vi "setMeasurement.vi"(1 "Measure":T1, 2 "Channel":T2) -> (0 "String":string)   [LabVIEW 2017]
uses:
  controls/Channel.ctl
  controls/Measure.ctl
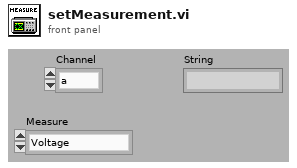
[diagram p1: front panel]
types:
  T1 = typedef "Measure.ctl" = enum16{"Voltage", "Current", "Resistance", "Power"}
  T2 = typedef "Channel.ctl" = enum16{"a", "b"}
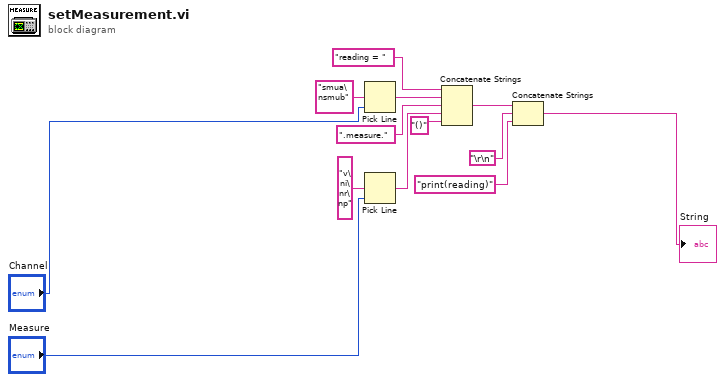
[diagram p0: block diagram]
diagram:
  n1 = Pick Line(multi-line string="smua\nsmub", line index="Channel") -> (output string=w13:string)  [unwired: 1 in]
  n2 = Pick Line(multi-line string="v\ni\nr\np", line index="Measure") -> (output string=w5:string)  [unwired: 1 in]
  n3 = Concatenate Strings("reading = ", w13, ".measure.", w5, "()") -> (w6:string)
  n4 = Concatenate Strings(w6, "\r\n", "print(reading)") -> (→"String":string)
